vi "load class.vi"(8 "error in":errorcluster, 9 "available class paths":path[](array[path]), 10 "available class names":string[](array[string]), 11 "Class Name":string) -> (0 "error out":errorcluster, 3 "Object Out":refnum<class>)   [LabVIEW 2013, in "class discovery singleton.lvlib"]
doc: "Attempts to load a class, by name, either from memory or from disk. First it tries the exact name in memory. Then it tries the filename on disk. Then it tries an approximate match of all VIs in memory."
uses:
  class discovery singleton.lvlib
  root configuration/TBM configuration.lvclass
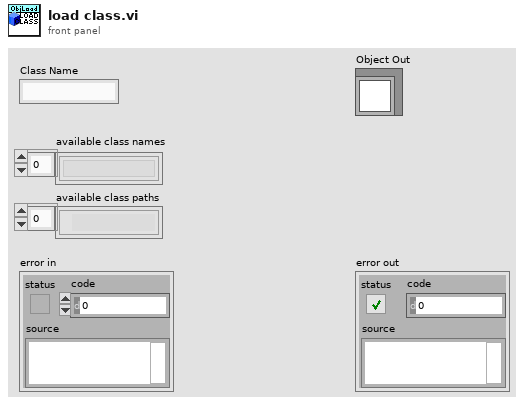
[diagram p1: front panel]
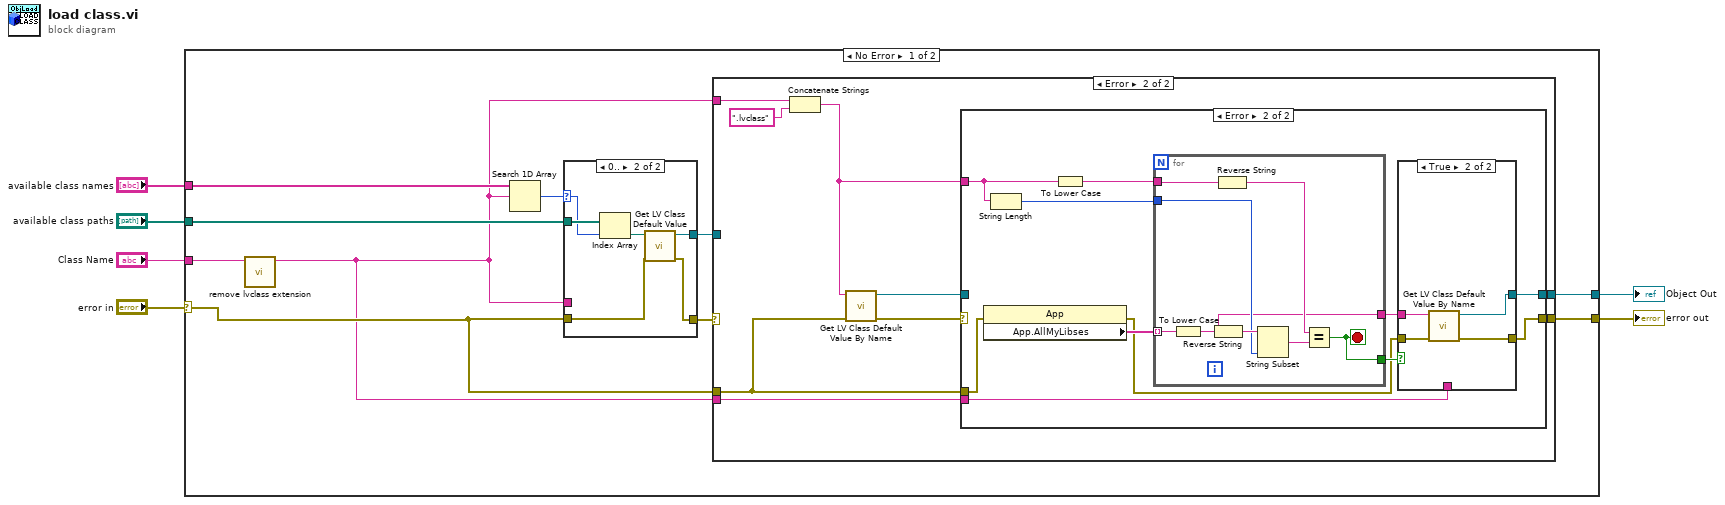
[diagram p0: block diagram]
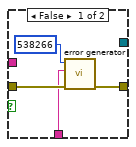
[diagram p4: hidden frame]
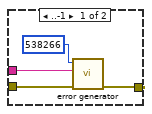
[diagram p5: hidden frame]
diagram:
  n1 = case shown="No Error" "error in" {
    selector: "error in" -> [w10 w67]
    tunnel: "Class Name" -> [w14 _]
    tunnel: [w13 _] -> w3
    tunnel: [w11 w67] -> w4
    tunnel: "available class paths" -> [w16 _]
    tunnel: "available class names" -> [w15 _]
    frame No Error {
      n2 = call "remove lvclass extension.vi"("class name in"=w14) -> ("class name out"=w7:string)  [unwired: 10 in]
      n3 = Search 1D Array(1D array=w15, element=w7) -> (index of element=w9:i32)  [unwired: 1 in]
      n4 = case shown="0.." w9 {
        selector: w9 -> [_ w62]
        tunnel: [w59 w66] -> w8
        tunnel: [_ w65] -> w12
        tunnel: w16 -> [_ w64]
        tunnel: w10 -> [w60 w61]
        tunnel: w7 -> [w57 _]
        frame ..-1 {
          n5 = call "error generator.vi"("error in"=w60, "append error message"=w57, "error code (0)"=538266) -> ("error out"=w59:errorcluster)  [unwired: 8 in]
        }
        frame 0.. {
          n6 = Index Array(array=w64, index=w62) -> (element=w63:path)
          n7 = call <vilib>:"Get LV Class Default Value.vi"("error in (no error)"=w61, "class path"=w63) -> ("error out"=w66:errorcluster, "object"=w65:refnum<class>)  [unwired: 8 in]
        }
      }
      n8 = case shown="Error" w8 {
        selector: w8 -> [w17 _]
        tunnel: [w18 w27] -> w13
        tunnel: w12 -> [w18 _]
        tunnel: [w17 w26] -> w11
        tunnel: w7 -> [_ w23]
        tunnel: w7 -> [_ w25]
        tunnel: w10 -> [_ w24]
        frame No Error {
        }
        frame Error {
          n9 = Concatenate Strings(w23, ".lvclass" ("string")) -> (w21:string)
          n10 = call <vilib>:"Get LV Class Default Value By Name.vi"("error in (no error)"=w24, "class name"=w21) -> ("error out"=w20:errorcluster, "object"=w19:refnum<class>)  [unwired: 8 in]
          n11 = case shown="Error" w20 {
            selector: w20 -> [w29 _]
            tunnel: [w28 w32] -> w27
            tunnel: [w29 w33] -> w26
            tunnel: w24 -> [_ w40]
            tunnel: w21 -> [_ w38]
            tunnel: w25 -> [_ w31]
            tunnel: w19 -> [w28 _]
            frame No Error {
            }
            frame Error {
              n12 = property class="App"(error in=w40) -> (error out=w34:errorcluster, "App.AllMyLibses"=w39:string[])  [unwired: 1 in, 1 out]
              n13 = String Length(string=w38) -> (length=w37:i32)
              n14 = To Lower Case(string=w38) -> (all lower case string=w30:string)
              n15 = for {
                tunnel: w39 -> [w51] mode=indexing
                tunnel: w30 -> [w56]
                tunnel: w37 -> [w54]
                tunnel: [w49] -> w36
                tunnel: [w50] -> w35
                stop <- w50 stop-if-true
                n16 = To Lower Case(string=w51) -> (all lower case string=w49:string)
                n17 = Reverse String(1:w49) -> (0:w55:string)
                n18 = Reverse String(1:w56) -> (0:w52:string)
                n19 = String Subset(string=w55, length (rest)=w54) -> (substring=w53:string)  [unwired: 1 in]
                n20 = Equal?(x=w52, y=w53) -> (x = y?=w50:bool)
              }
              n21 = case shown="True" w35 {
                tunnel: w36 -> [_ w48]
                tunnel: w34 -> [w42 w47]
                tunnel: [w43 w46] -> w33
                tunnel: [_ w45] -> w32
                tunnel: w31 -> [w41 _]
                frame False {
                  n22 = call "error generator.vi"("error in"=w42, "append error message"=w41, "error code (0)"=538266) -> ("error out"=w43:errorcluster)  [unwired: 8 in]
                }
                frame True {
                  n23 = call <vilib>:"Get LV Class Default Value By Name.vi"("error in (no error)"=w47, "class name"=w48) -> ("error out"=w46:errorcluster, "object"=w45:refnum<class>)  [unwired: 8 in]
                }
              }
            }
          }
        }
      }
    }
    frame Error {
    }
  }
  "error out" <- w4
  "Object Out" <- w3
